vi "user32_DispatchMessage.vi"(8 "错误输入（无错误）":errorcluster, 11 "lpMsg":u32) -> (0 "错误输出":errorcluster, 3 "dup lpMsg":u32)   [LabVIEW 2011]
doc: "该函数分发一个消息给窗口程序。通常消息从GetMessage函数获得。消息被分发到回调函数（过程函数)，作用是消息传递给操作系统，然后操作系统去调用我们的回调函数，也就是说我们在窗体的过程函数中处理消息。"
uses:
  user32.dll
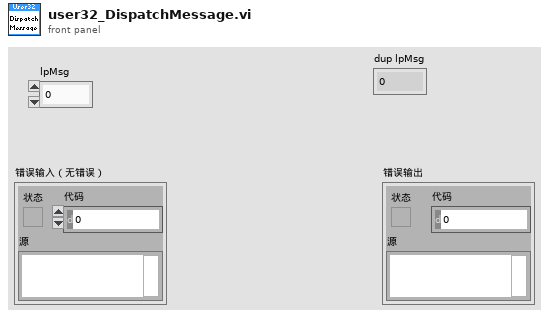
[diagram p1: front panel]
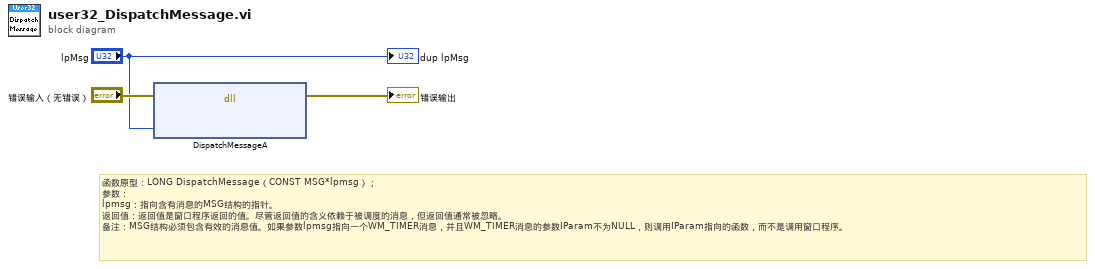
[diagram p0: block diagram]
diagram:
  # "函数原型：LONG DispatchMessage（CONST MSG*lpmsg）；\n参数：\nlpmsg：指向含有消息的MSG结构的指针。\n返回值：返回值是窗口程序返回的值。尽管返回值的含义依赖于被调度的消息，但返回值通常被忽略。\n备注：MSG结构必须包含有效的消息值。如果参数lpmsg指向一个WM_TIMER消息，并且WM_TIMER消息的参数IParam不为NULL，则调用IParam指向的函数，而不是调用窗口程序。"
  n1 = dll-call lib="user32.dll" fn="DispatchMessageA"(error in="错误输入（无错误）", "lpMsg"="lpMsg") -> (error out=→"错误输出":errorcluster)  [unwired: 4 in, 1 out]
  "dup lpMsg" <- "lpMsg"
